vi "ALTS-2015 Check for UUT Clamped and Select Test.vi"(8 "error in":errorcluster, 10 "Test Type In":i32, 11 "Station Cluster":T1) -> (0 "error out":errorcluster)   [LabVIEW 2013]
doc: "Copyright © 2005, Soliton Technologies.\nAll rights reserved."
uses:
  Controls/ALTS-2015 Station Cluster.ctl
  Controls/ALTS-2015 Status Message Options.ctl
  Controls/ALTS-2015 LV2GBL Station Info Options.ctl
  Controls/ALTS-2015 Ring Indicator Enum.ctl
  Controls/ALTS-2015 Status Ring Indicator.ctl
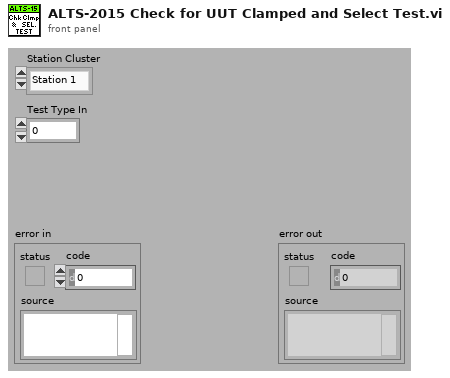
[diagram p1: front panel]
types:
  T1 = typedef "ALTS-2015 Station Cluster.ctl" = enum16{"Station 1", "Station 2", "Station 3", "Station 4"}
  T2 = typedef "ALTS-2015 Status Message Options.ctl" = enum16{"Initializing...", "Enter User Login...", "Enter Work Order Number...", "Enter Serial Number...", "Valid Serial Number...", "Invalid Serial Number...", "Start Tag Received...", "Stop Tag Received...", "UUT Clamped...", "UUT not Clamped...", "Test Running...", "Test Complete...", "Writing Result to DB...", "DB Entry Pressed...", "Clearing Serial Number...", "Idle...", "Exiting..."}
  T3 = typedef "ALTS-2015 LV2GBL Station Info Options.ctl" = enum16{"Init", "Read", "Read All", "Write Sensor ID", "Write  Work Order", "Write Serial Number", "Write Test Data", "Write Station Status", "Write Station Occupancy", "Write Station Test Type", "Write Rerun", "Clear All", "Clear Test Result"}
  T4 = typedef "ALTS-2015 Status Ring Indicator.ctl" = u16
  T5 = typedef "ALTS-2015 Ring Indicator Enum.ctl" = enum16{"Idle", "Test Running", "Unit Clamped", "Unit not Clamped", "Pass", "Fail"}
  T6 = typedef "ALTS-2015 Station Details.ctl" = cluster{"Station Number":string, "Work Order Number":string, "Sensor Name":string, "Pressure (PSI)":string, "Flow (SCCM)":string, "Test Time ":string, "Test Result":string, "Serial Number":string, "Station Status":T4, "Station Occupied?":bool, "Rerun Count":i32, "Test Type":i32}
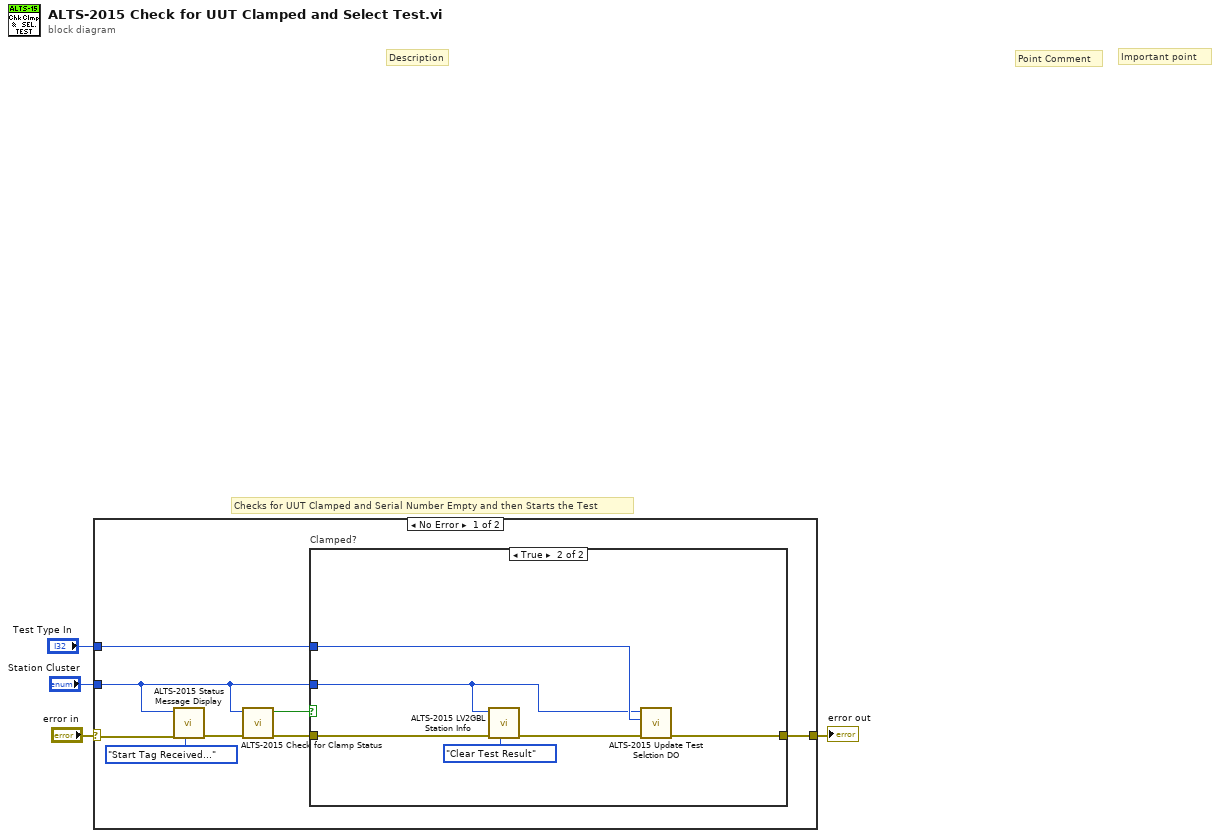
[diagram p0: block diagram]
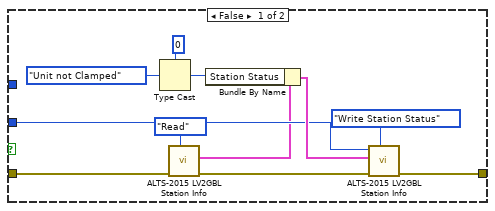
[diagram p2: hidden frame]
diagram:
  # "Checks for UUT Clamped and Serial Number Empty and then Starts the Test"
  # "Point Comment"
  # "Important point"
  # "Description"
  n1 = case shown="No Error" "error in" {
    selector: "error in" -> [w8 w30]
    tunnel: [w7 w30] -> w3
    tunnel: "Station Cluster" -> [w6 _]
    tunnel: "Test Type In" -> [w5 _]
    frame No Error {
      n2 = call "ALTS-2015 Status Message Display.vi"("Status Message Options"=ALTS-2015_Status_Message_Options."Start Tag Received...", "error in (no error)"=w8, "Station Enum"=w6) -> ("error out"=w9:errorcluster)  [unwired: 7 in, 1 out]
      n3 = call "ALTS-2015 Check for Clamp Status .vi"("error in (no error)"=w9, "Station Cluster"=w6) -> ("error out"=w12:errorcluster, "Clamp?"=w11:bool)  [unwired: 8 in]
      n4 = case "Clamped?" shown="True" w11 {
        tunnel: w12 -> [w15 w28]
        tunnel: [w20 w29] -> w7
        tunnel: w6 -> [w21 w26]
        tunnel: w5 -> [_ w27]
        frame False {
          n5 = Type Cast(type=T4 0 ("Station Status"), x=ALTS-2015_Ring_Indicator_Enum."Unit not Clamped" ("Ring Indicator Options")) -> (*(type *) &x=w17:T4)
          n6 = call "ALTS-2015 LV2GBL Station Info.vi"("Options"=ALTS-2015_LV2GBL_Station_Info_Options."Read", "error in"=w15) -> ("error out"=w14:errorcluster, "Station Details"=w13:T6)  [unwired: 7 in, 1 out]
          n7 = Bundle By Name(cluster=w13, "Station Status"=w17) -> (w22:T6)
          n8 = call "ALTS-2015 LV2GBL Station Info.vi"("Options"=ALTS-2015_LV2GBL_Station_Info_Options."Write Station Status", "error in"=w14, "Station"=w22, "Station Cluster"=w21) -> ("error out"=w20:errorcluster)  [unwired: 5 in, 2 out]
        }
        frame True {
          n9 = call "ALTS-2015 LV2GBL Station Info.vi"("Options"=ALTS-2015_LV2GBL_Station_Info_Options."Clear Test Result", "error in"=w28, "Station Cluster"=w26) -> ("error out"=w24:errorcluster)  [unwired: 6 in, 2 out]
          n10 = call "ALTS-2015 Update Test Selction DO.vi"("error in"=w24, "Test Type In"=w27, "Station Cluster"=w26) -> ("error out"=w29:errorcluster)  [unwired: 8 in]
        }
      }
    }
    frame Error {
    }
  }
  "error out" <- w3
